vi "Create Execution Unit.vi"(8 "error in":errorcluster, 10 "Item Ref":T2=18446744073709551615 format="%.0x", 11 "Execution Unit Factory Implementation in":refnum<class "Execution Unit Factory.lvclass">) -> (0 "error out":errorcluster, 1 "Asynchronous Execution Units":T1[](array[typedef]) {"ReadWrite Channels" format="%.0x"; "Outgoing Channels" format="%.0x"; "Incoming Channels" format="%.0x"}, 2 "Inline Execution Units":T1[](array[typedef]) {"ReadWrite Channels" format="%.0x"; "Outgoing Channels" format="%.0x"; "Incoming Channels" format="%.0x"}, 3 "Execution Unit Factory Implementation out":refnum<class "Execution Unit Factory.lvclass">)   [LabVIEW 2020, in "AIM ARINC 429 Engine.lvlib" / "Implementation.lvlib" / "Execution Unit Factory.lvclass"]
uses:
  Execution Unit Factory.lvclass
  <vilib>/NI VeriStand/Custom Device API/Custom Device Item Ref.ctl
  Interfaces/Controls/Execution Unit Information.ctl
  Interfaces/Execution Unit/Execution Unit.lvclass
  Execution Unit/Execution Unit.lvclass
  C:/Users/nitest/Desktop/Git 2020/niveristand-aim-arinc429-custom-device/Source/Custom Device Support/Engine/Interfaces/Execution Unit/Execution Unit.lvclass
  Rx Execution Unit/Rx Execution Unit.lvclass
  Logging Execution Unit/Logging Execution Unit.lvclass
  Tx Scheduled Labels Execution Unit/Tx Scheduled Labels Execution Unit.lvclass
  C:/Users/nitest/Desktop/Git 2020/niveristand-aim-arinc429-custom-device/Source/Custom Device Support/Engine/Implementation/Execution Unit/Execution Unit.lvclass
  Tx Acyclic Labels Execution Unit/Tx Acyclic Labels Execution Unit.lvclass
  <vilib>/NI VeriStand/Custom Device API/Custom Device API.lvlib
  Interfaces/Interfaces.lvlib
  System Explorer/Implementation/Implementation.lvlib
  Scripting/AIM/AIM ARINC 429 Scripting.lvlib
  C:/Users/nitest/Desktop/Git 2020/niveristand-aim-arinc429-custom-device/Source/Custom Device Support/Engine/Implementation/Rx Execution Unit/Rx Execution Unit.lvclass
  C:/Users/nitest/Desktop/Git 2020/niveristand-aim-arinc429-custom-device/Source/Custom Device Support/Engine/Implementation/Logging Execution Unit/Logging Execution Unit.lvclass
  C:/Users/nitest/Desktop/Git 2020/niveristand-aim-arinc429-custom-device/Source/Custom Device Support/Engine/Implementation/Tx Scheduled Labels Execution Unit/Tx Scheduled Labels Execution Unit.lvclass
  C:/Users/nitest/Desktop/Git 2020/niveristand-aim-arinc429-custom-device/Source/Custom Device Support/Engine/Implementation/Tx Acyclic Labels Execution Unit/Tx Acyclic Labels Execution Unit.lvclass
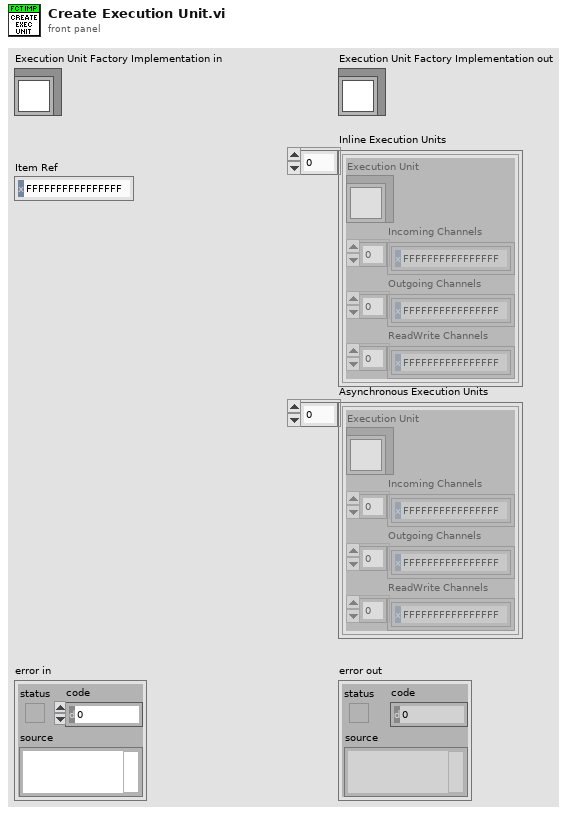
[diagram p1: front panel]
types:
  T1 = typedef "AIM ARINC 429 Engine.lvlib/Interfaces.lvlib/Execution Unit Information.ctl" = cluster{"Execution Unit":refnum<class "Execution Unit.lvclass">, "Incoming Channels":T2[], "Outgoing Channels":T2[], "ReadWrite Channels":T2[]}
  T2 = typedef "Custom Device API.lvlib/Custom Device Item Ref.ctl" = u64
  T3 = typedef "RT Hardware Channel Settings.ctl" = cluster{"channel #":u16, "channel handle":u64, "labels settings for RT":T4[], "speed":T11}
  T4 = typedef "RT Label Settings.ctl" = cluster{"Name":string, "xmlName":string, "label":T5, "transfer period":u32, "SDI_Enabled":bool, "SDI":u8, "parameter driver data":T6, "transfer type":T9, "has timestamp?":bool, "Label Disable/Trigger Channel Reference":T2, "Message Handle":u64, "Initialized?":bool, "Word Initial Raw Value":u32, "Label Timestamp Channel Data Reference":T10, "disabled":bool}
  T5 = typedef "Label.ctl" = u8
  T6 = typedef "RT Parameters.ctl" = cluster{"parameter definitions":T7[], "Tx parameter refs":T2[]}
  T7 = typedef "Parameter Definition.ctl" = cluster{"start index":i32, "size":i32, "encoding":T8, "signed":bool, "scale multiplier":dbl, "scale offset":dbl, "default value":dbl}
  T8 = typedef "Encoding and Decoding.lvlib/Encoding.ctl" = enum16{"BNR", "BCD", "Discrete"}
  T9 = typedef "Transfer Type.ctl" = enum16{"Scheduled", "Acyclic", "Block", "Strobe"}
  T10 = typedef "Custom Device API.lvlib/Data Reference.ctl" = i32
  T11 = typedef "Transfer Speed.ctl" = enum16{"LO (12.5 kb/s)", "HI (100 kb/s)"}
  T12 = cluster{"transfer type":T9, "Name":string, "hardware channel data":T3[], "Outgoing Channels":T2[], "ReadWrite Channels":T2[]}[]
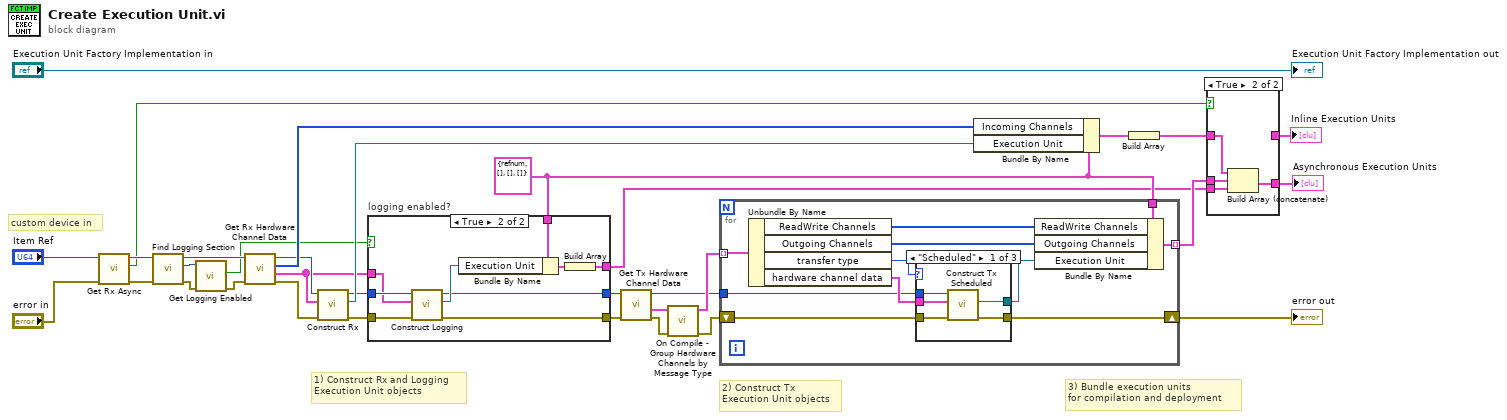
[diagram p0: block diagram]
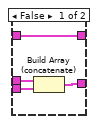
[diagram p2: hidden frame]
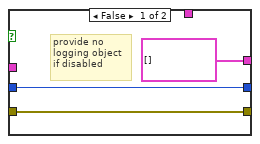
[diagram p3: hidden frame]
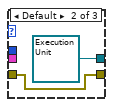
[diagram p4: hidden frame]
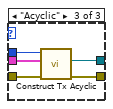
[diagram p5: hidden frame]
diagram:
  w14 = T1 {"Execution Unit"=refnum, "Incoming Channels"=[], "Outgoing Channels"=[], "ReadWrite Channels"=[]} ("Execution Unit Information")
  # "2) Construct Tx\nExecution Unit objects"
  # "custom device in"
  # "3) Bundle execution units\nfor compilation and deployment"
  # "1) Construct Rx and Logging\nExecution Unit objects"
  n1 = call "Get Rx Async.vi"("error in"="error in", "custom device ref"="Item Ref") -> ("error out"=w7:errorcluster, "Rx Async?"=w3:bool, "custom device ref out"=w6:T2)  [unwired: 7 in]
  n2 = call "Find Logging Section.vi"("error in"=w7, "custom device ref"=w6) -> ("error out"=w12:errorcluster, "logging"=w11:T2, "custom device ref out"=w9:T2)  [unwired: 7 in]
  n3 = call "Get Logging Enabled.vi"("error in"=w12, "logging ref"=w11) -> ("error out"=w10:errorcluster, "logging enabled"=w8:bool)  [unwired: 7 in, 1 out]
  n4 = call "Get Rx Hardware Channel Data.vi"("error in"=w10, "custom device ref in"=w9) -> ("error out"=w29:errorcluster, "Rx hardware channel data"=w18:T3[], "incoming channels"=w30:T2[], "custom device ref out"=w22:T2)  [unwired: 6 in]
  n5 = call "Construct Rx.vi"("error in"=w29, "Rx hardware channels in"=w18, "custom device ref in"=w22) -> ("error out"=w19:errorcluster, "Rx Execution Unit out"=w23:refnum<class "Rx Execution Unit.lvclass">, "custom device ref out"=w20:T2)  [unwired: 6 in]
  n6 = case "logging enabled?" shown="True" w8 {
    tunnel: w20 -> [w35 w45]
    tunnel: w19 -> [w34 w44]
    tunnel: w18 -> [_ w43]
    tunnel: [w35 w41] -> w17
    tunnel: [w34 w40] -> w16
    tunnel: w14 -> [_ w38]
    tunnel: [T1[] [] w37] -> w13
    frame False {
      # "provide no\nlogging object\nif disabled"
    }
    frame True {
      n7 = call "Construct Logging.vi"("error in"=w44, "Logging hardware channels in"=w43, "custom device ref in"=w45) -> ("error out"=w40:errorcluster, "Logging Execution Unit out"=w42:refnum<class "Logging Execution Unit.lvclass">, "custom device ref out"=w41:T2)  [unwired: 6 in]
      n8 = Bundle By Name(cluster=w38, "Execution Unit"=w42) -> (w39:T1)
      n9 = Build Array(w39) -> (w37:T1[])
    }
  }
  n10 = call "Get Tx Hardware Channel Data.vi"("error in"=w16, "custom device ref in"=w17) -> ("error out"=w28:errorcluster, "Tx hardware channel data"=w27:T3[], "custom device ref out"=w21:T2)  [unwired: 6 in, 1 out]
  n11 = call "On Compile - Group Hardware Channels by Message Type.vi"("error in"=w28, "hardware channel data"=w27) -> ("error out"=w25:errorcluster, "hardware channel data by transfer type"=w26:T12)  [unwired: 8 in]
  n12 = for {
    tunnel: w14 -> [w55]
    tunnel: [w56] -> w32 mode=indexing
    tunnel: w26 -> [w54] mode=indexing
    shift-right: [w47] -> w24
    shift-left: w25 -> [w48]
    tunnel: w21 -> [w46]
    n13 = Unbundle By Name(w54) -> ("ReadWrite Channels"=w53:T2[], "Outgoing Channels"=w52:T2[], "transfer type"=w51:T9, "hardware channel data"=w50:T3[])
    n14 = case shown="\"Scheduled\"" w51 {
      tunnel: w50 -> [w59 _ w66]
      tunnel: [w58 refnum<class "Execution Unit.lvclass"> refnum ("Communication Bus Template Interfaces:Implementation.lvlib:Execution Unit.lvclass") w65] -> w49
      tunnel: w48 -> [w61 w62 w68]
      tunnel: [w60 w62 w67] -> w47
      tunnel: w46 -> [w57 _ w64]
      frame "Scheduled" {
        n15 = call "Construct Tx Scheduled.vi"("error in"=w61, "Tx Scheduled hardware channels in"=w59, "custom device ref in"=w57) -> ("error out"=w60:errorcluster, "Tx Scheduled Execution Unit out"=w58:refnum<class "Tx Scheduled Labels Execution Unit.lvclass">)  [unwired: 6 in, 1 out]
      }
      frame Default {
      }
      frame "Acyclic" {
        n16 = call "Construct Tx Acyclic.vi"("error in"=w68, "Tx Acyclic hardware channels in"=w66, "custom device ref in"=w64) -> ("error out"=w67:errorcluster, "Tx Acyclic Execution Unit out"=w65:refnum<class "Tx Acyclic Labels Execution Unit.lvclass">)  [unwired: 6 in, 1 out]
      }
    }
    n17 = Bundle By Name(cluster=w55, "ReadWrite Channels"=w53, "Outgoing Channels"=w52, "Execution Unit"=w49) -> (w56:T1)
  }
  "error out" <- w24
  n18 = Bundle By Name(cluster=w14, "Incoming Channels"=w30, "Execution Unit"=w23) -> (w31:T1)
  n19 = Build Array(w31) -> (w2:T1[])
  n20 = case shown="True" w3 {
    tunnel: w32 -> [w72 w76]
    tunnel: [w70 w75] -> w15
    tunnel: w13 -> [w71 w74]
    tunnel: w2 -> [w69 w73]
    tunnel: [w69 _] -> w1
    frame False {
      n21 = Build Array (concatenate)(w72, w71) -> (w70:T1[])
    }
    frame True {
      n22 = Build Array (concatenate)(w73, w76, w74) -> (w75:T1[])
    }
  }
  "Inline Execution Units" <- w1
  "Asynchronous Execution Units" <- w15
  "Execution Unit Factory Implementation out" <- "Execution Unit Factory Implementation in"
